vi "Colorbar1001.vi"   [LabVIEW 2013]
uses:
  <vilib>/Heliosphere Research LLC/Advanced Plotting Toolkit/Advanced Plotting Toolkit.lvlib
types:
  T1 = typedef "Advanced Plotting Toolkit.lvlib/PlotID.ctl" = i32
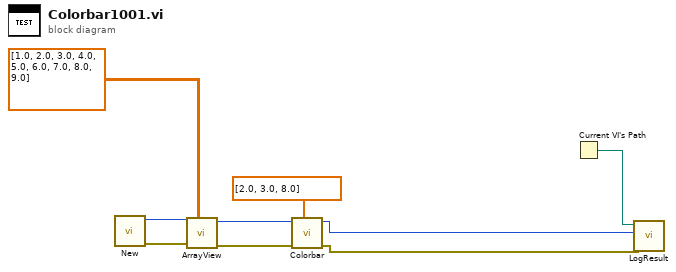
[diagram p0: block diagram]
diagram:
  n1 = call <vilib>:"New.vi"() -> ("error out"=w8:errorcluster, "Plot ID"=w7:T1)  [unwired: 10 in]
  n2 = call <vilib>:"ArrayView.vi"("Data"=dbl[][] [[1.0, 2.0, 3.0], [4.0, 5.0, 6.0], [7.0, 8.0, 9.0]], "error in (no error)"=w8, "Plot ID"=w7) -> ("error out"=w4:errorcluster, "Plot ID Out"=w5:T1)  [unwired: 7 in]
  n3 = call <vilib>:"Colorbar.vi"("Ticks"=dbl[] [2.0, 3.0, 8.0], "error in (no error)"=w4, "Plot ID"=w5) -> ("error out"=w3:errorcluster, "Plot ID Out"=w2:T1)  [unwired: 7 in]
  n4 = Current VI's Path() -> (path=w9:path)
  n5 = call "LogResult.vi"("Test Result"=w3, "Test Artifact"=w2, "VI Path"=w9) -> ()  [unwired: 9 in]
